vi "FTW-Time-Now.vi"(0 "Previous Time":dbl format="%^<%Y-%m-%dT%H:%M:%S%3uZ>T", 11 "error in":errorcluster) -> (4 "Current Time":dbl format="%^<%Y-%m-%dT%H:%M:%S%3uZ>T", 6 "Elapsed Time":dbl format="%.6fsec", 15 "error out":errorcluster)   [LabVIEW 2015]
panel:
  # "Inputs"
  # "Outputs"
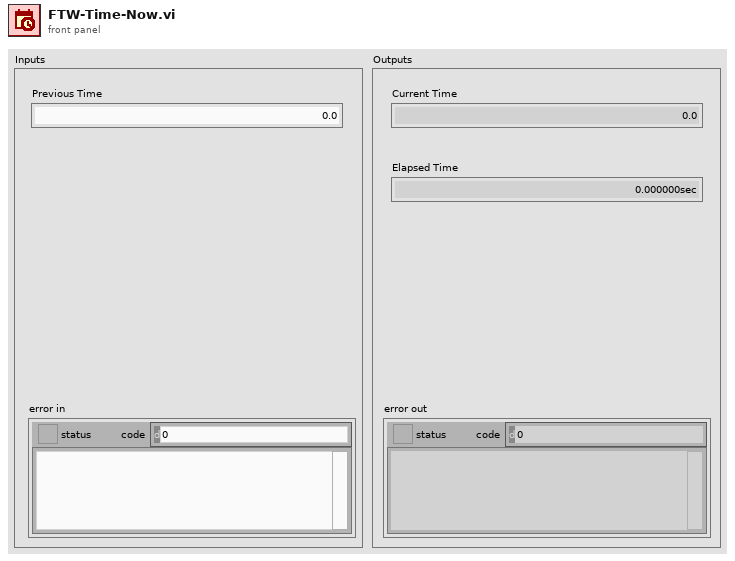
[diagram p1: front panel]
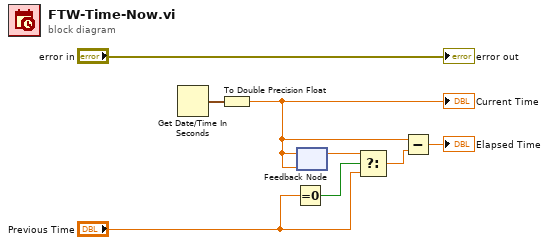
[diagram p0: block diagram]
diagram:
  n1 = Get Date/Time In Seconds() -> (seconds since 1Jan1904=w3:timestamp)
  n2 = To Double Precision Float(number=w3) -> (double precision float=w2:dbl)
  "Current Time" <- w2
  n3 = Equal To 0?(x="Previous Time") -> (x = 0?=w5:bool)
  n4 = feedback-in #1(w2) -> ()
  n5 = feedback #1(w2) -> (w7:dbl)
  n6 = Select(t=w7, s=w5, f="Previous Time") -> (s? t:f=w1:dbl)
  n7 = Subtract(x=w2, y=w1) -> (x-y=→"Elapsed Time":dbl)
  "error out" <- "error in"
